vi "get_components.vi"(8 "error in (no error)":errorcluster, 11 "SpaceVector in":refnum<class "SpaceVector.lvclass">) -> (0 "error out":errorcluster, 1 "x":dbl[unit], 2 "x/y/z":T1, 3 "SpaceVector out":refnum<class "SpaceVector.lvclass">, 4 "z":dbl[unit], 6 "y":dbl[unit])   [LabVIEW 2010, in "SpaceVector.lvclass"]
uses:
  SpaceVector.lvclass
  arrays/space_vector_array.ctl
  SpaceVector.lvclass/SpaceVector.ctl
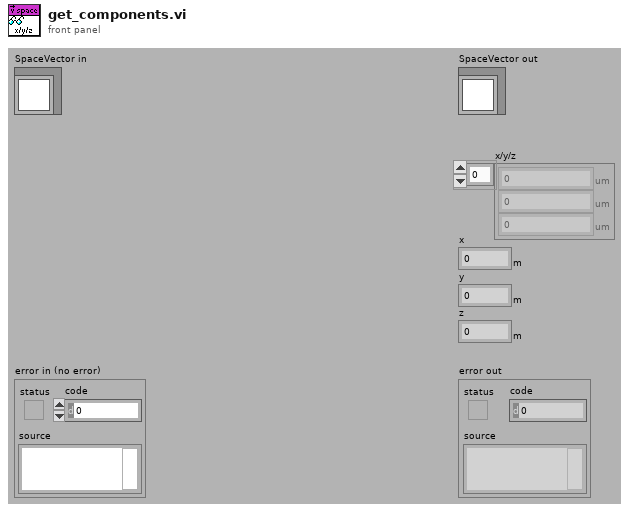
[diagram p1: front panel]
types:
  T1 = typedef "space_vector_array.ctl" = dbl[unit][]
  T2 = cluster{"space vector[0]":dbl[unit], "space vector[1]":dbl[unit], "space vector[2]":dbl[unit]}
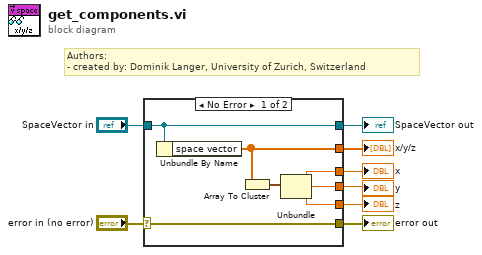
[diagram p0: block diagram]
diagram:
  # "Authors: \n- created by: Dominik Langer, University of Zurich, Switzerland"
  n1 = case shown="No Error" "error in (no error)" {
    selector: "error in (no error)" -> [w15 w17]
    tunnel: [w15 w17] -> w7
    tunnel: [w14 w16] -> w5
    tunnel: "SpaceVector in" -> [w14 w16]
    tunnel: [w13 _] -> w4
    tunnel: [w11 _] -> w2
    tunnel: [w10 _] -> w1
    tunnel: [w9 _] -> w3
    frame No Error {
      n2 = Unbundle By Name(w14) -> ("space vector"=w13:T1)
      n3 = Array To Cluster(array=w13) -> (cluster=w12:T2)
      n4 = Unbundle(w12) -> ("space vector[0]"=w11:dbl[unit], "space vector[1]"=w10:dbl[unit], "space vector[2]"=w9:dbl[unit])
    }
    frame Error {
    }
  }
  "error out" <- w7
  "SpaceVector out" <- w5
  "x/y/z" <- w4
  "z" <- w3
  "x" <- w2
  "y" <- w1
